vi "Extract Becker-Hickl Format String.vi"(11 "String in":string) -> (3 "Format String":string)   [LabVIEW 2021, in "Becker-Hickl Files.lvlib"]
uses:
  Becker-Hickl Files.lvlib
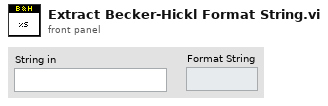
[diagram p1: front panel]
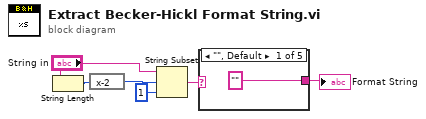
[diagram p0: block diagram]
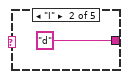
[diagram p2: hidden frame]
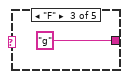
[diagram p3: hidden frame]
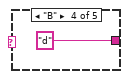
[diagram p4: hidden frame]
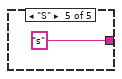
[diagram p5: hidden frame]
diagram:
  n1 = String Length(string="String in") -> (length=w4:i32)
  n2 = expression code="x-2"(w4) -> (w3:i32)
  n3 = String Subset(string="String in", offset (0)=w3, length (rest)=1 ("length (rest)")) -> (substring=w2:string)
  n4 = case shown="\"\", Default" w2 {
    tunnel: ["" ("Format String") "d" ("Format String") "g" ("Format String") "d" ("Format String") "s" ("Format String")] -> w1
    frame "", Default {
    }
    frame "I" {
    }
    frame "F" {
    }
    frame "B" {
    }
    frame "S" {
    }
  }
  "Format String" <- w1
